vi "Launch Async Force config.vi"() -> ()   [LabVIEW 2021]
uses:
  Options.ctl
panel:
  in  "Launcher":i32=1 min=1 step=1
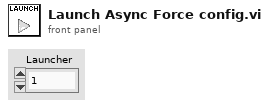
[diagram p1: front panel]
types:
  T1 = typedef "Options.ctl" = u16
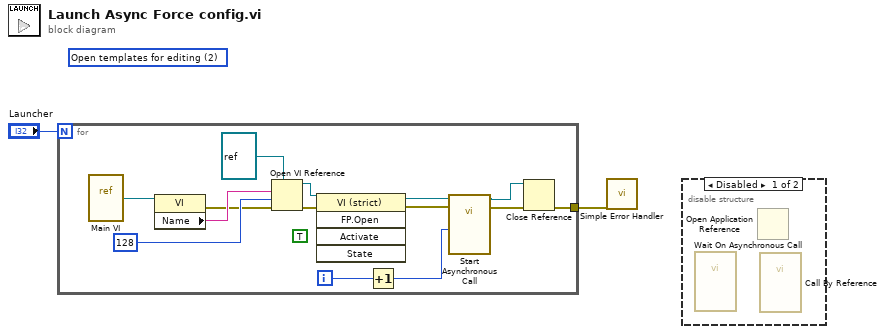
[diagram p0: block diagram]
diagram:
  (unwired) T1 2 items=["Record modifications"=1, "Open templates for editing"=2] ("Ring")
  n1 = for {
    N: "Launcher" -> [_]
    tunnel: [w10] -> w1
    i -> [w8]
    (unwired) TRUE ("Activate?")
    n2 = vi-ref "Main VI.vi"() -> (w16:refnum<vi>)
    n3 = property class="VI"(reference=w16) -> (error out=w13:errorcluster, "Name"=w14:string)  [unwired: 1 in, 1 out]
    n4 = Open VI Reference(type specifier VI Refnum (for type only)=refnum<vi> refnum, vi path=w14, options=128, error in (no error)=w13) -> (vi reference=w6:refnum<vi>, error out=w7:errorcluster)  [unwired: 2 in]
    n5 = invoke class="VI (strict)" method="FP.Open"(reference=w6, error in=w7) -> (reference out=w4:refnum<vi>, error out=w5:errorcluster)  [unwired: 3 in, 3 out]
    n6 = Increment(x=w8) -> (x+1=w3:i32)
    n7 = call-by-ref "Start Asynchronous Call"(reference=w4, error in=w5, "Numeric"=w3) -> (reference out=w11:refnum<vi>, error out=w12:errorcluster)  [unwired: 11 in]
    n8 = Close Reference(reference=w11, error in (no error)=w12) -> (error out=w10:errorcluster)
  }
  n9 = call <vilib>:"Simple Error Handler.vi"("error in (no error)"=w1) -> ()  [unwired: 4 in, 5 out]
  n10 = disable-structure shown="Disabled" {
    frame Disabled {
      n11 = call-by-ref "Wait On Asynchronous Call"() -> ()  [unwired: 2 in, 2 out]
      n12 = Open Application Reference() -> ()  [unwired: 4 in, 2 out]
      n13 = call-by-ref "?"() -> ()  [unwired: 2 in, 2 out]
    }
    frame Enabled {
    }
  }
